vi "Start Sync.vi"(8 "error in":errorcluster, 11 "gRPC service in":refnum<class "ServiceBase.lvclass">) -> (0 "error out":errorcluster, 3 "gRPC service out":refnum<class "ServiceBase.lvclass">)   [LabVIEW 2019, in "gRPC-servicer.lvlib" / "ServiceBase.lvclass"]
uses:
  ServiceBase.lvclass
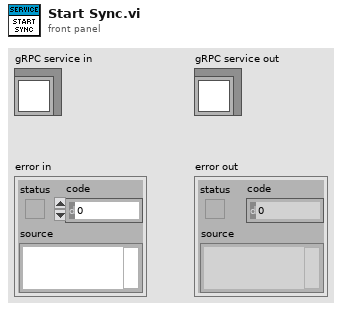
[diagram p1: front panel]
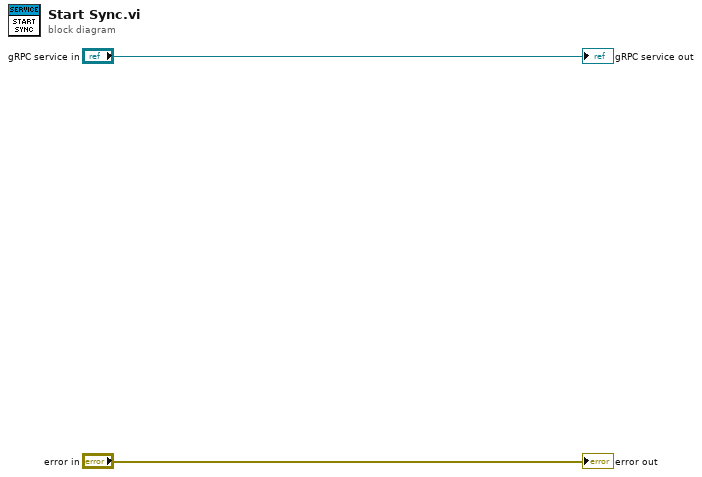
[diagram p0: block diagram]
diagram:
  "error out" <- "error in"
  "gRPC service out" <- "gRPC service in"
